vi "UV_SendCMD.vi"(6 "delay(ms)":i32=50, 7 "timeout(ms)":i32=500, 8 "error in":errorcluster, 9 "value":string, 10 "function":string, 11 "VISA resource name":refnum<visa-resource-name>) -> (0 "error out":errorcluster, 1 "response":string, 3 "VISA resource name out":refnum<visa-resource-name>)   [LabVIEW 2018]
uses:
  convert/NUM U8_ASCII (SubVI).vi
  convert/CMD_SUM (SubVI).vi
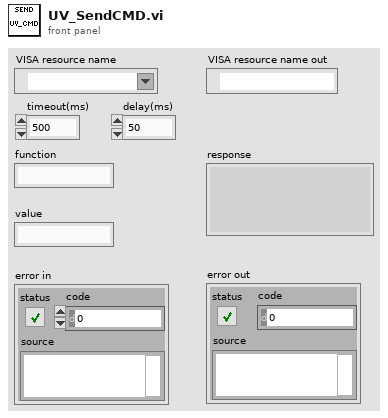
[diagram p1: front panel]
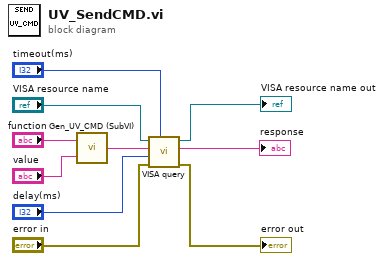
[diagram p0: block diagram]
diagram:
  n1 = call "Gen_UV_CMD (SubVI).vi"("value"="value", "function"="function") -> ("commu_data"=w10:string)
  n2 = call "VISA query.vi"("timeout(ms)"="timeout(ms)", "error in"="error in", "delay(ms)"="delay(ms)", "write buffer"=w10, "VISA resource name"="VISA resource name") -> ("error out"=→"error out":errorcluster, "read buffer"=→"response":string, "VISA resource name out"=→"VISA resource name out":refnum<visa-resource-name>)  [unwired: 4 in]
